vi "init.vi"(8 "error in (no error)":errorcluster, 9 "SwapBytes":bool, 10 "Size":i32, 11 "U8ArrayBuilderManualIndexing in":refnum<class "U8ArrayBuilderManualIndexing.lvclass">) -> (0 "error out":errorcluster, 3 "U8ArrayBuilderManualIndexing out":refnum<class "U8ArrayBuilderManualIndexing.lvclass">)   [LabVIEW 2016, in "RTUtilities.lvlib" / "U8ArrayBuilderManualIndexing.lvclass"]
uses:
  U8ArrayBuilderManualIndexing.lvclass
  U8ArrayBuilderManualIndexing.lvclass/U8ArrayBuilderManualIndexing.ctl
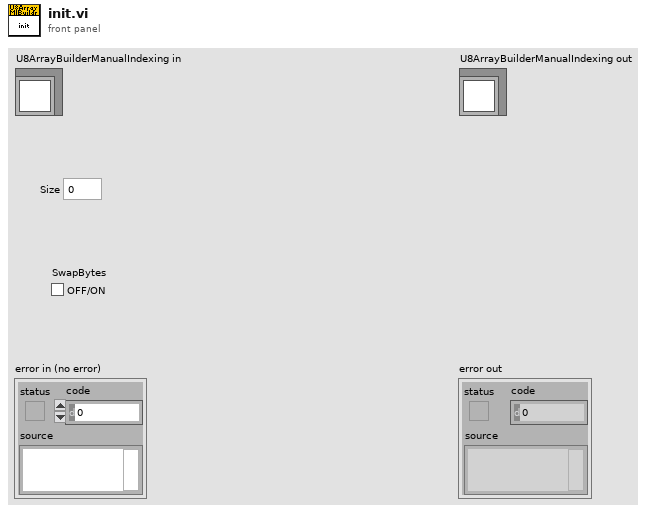
[diagram p1: front panel]
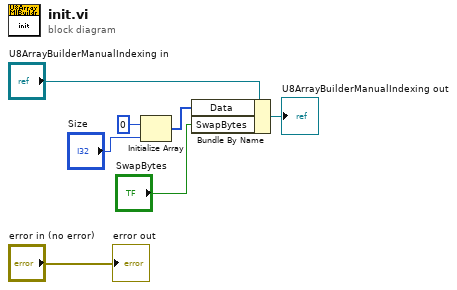
[diagram p0: block diagram]
diagram:
  n1 = Initialize Array(u8 0 ("element"), "Size") -> (w2:u8[])
  n2 = Bundle By Name(cluster="U8ArrayBuilderManualIndexing in", "Data"=w2, "SwapBytes"="SwapBytes") -> (→"U8ArrayBuilderManualIndexing out":refnum<class "U8ArrayBuilderManualIndexing.lvclass">)
  "error out" <- "error in (no error)"
